vi "加标回收启动对话框.vi"(11 "测试模式":enum16{"水样测试", "平行样测试", "加标回收", "集成干预测试"}(ring)) -> (1 "流程参数":T1, 2 "启动参数":T2, 3 "check ？":bool)   [LabVIEW 2016, in "质控单元V4.lvlib"]
panel:
  in  "氟化物":bool caption="启用"
  in  "采配水":bool=TRUE
  in  "取消":bool
  in  "确认":bool
  in  "CODCr":bool caption="启用"
  in  "CODMn":bool caption="启用"
  in  "总氮":bool caption="启用"
  in  "总磷":bool caption="启用"
  in  "氨氮":bool caption="启用"
  # "请选择启动参数和流程"
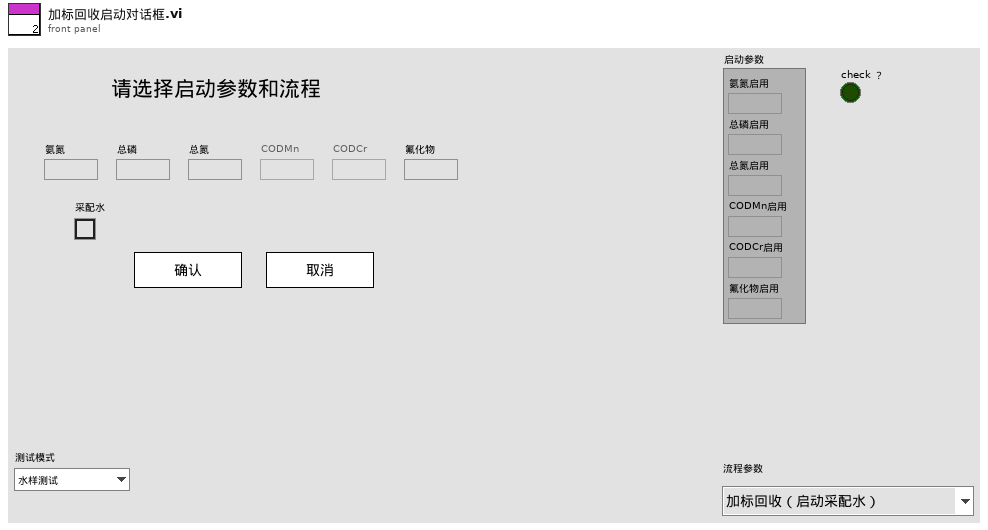
[diagram p1: front panel]
types:
  T1 = typedef "质控单元V4.lvlib/测试流程.ctl" = enum16{"加标回收（启动采配水）", "加标回收（不启动采配水）", "水样测试（启动采配水）", "水样测试（不启动采配水）", "平行样测试（启动采配水）", "平行样测试（不启动采配水）", "集成干预测试"}
  T2 = typedef "质控单元V4.lvlib/启动参数.ctl" = cluster{"氨氮启用":bool, "总磷启用":bool, "总氮启用":bool, "CODMn启用":bool, "CODCr启用":bool, "氟化物启用":bool}
  T3 = cluster{"氨氮":bool, "总磷":bool, "总氮":bool, "CODMn":bool, "CODCr":bool, "氟化物":bool}
  T4 = enum8{"Enabled", "Disabled", "Disabled and Grayed Out"}
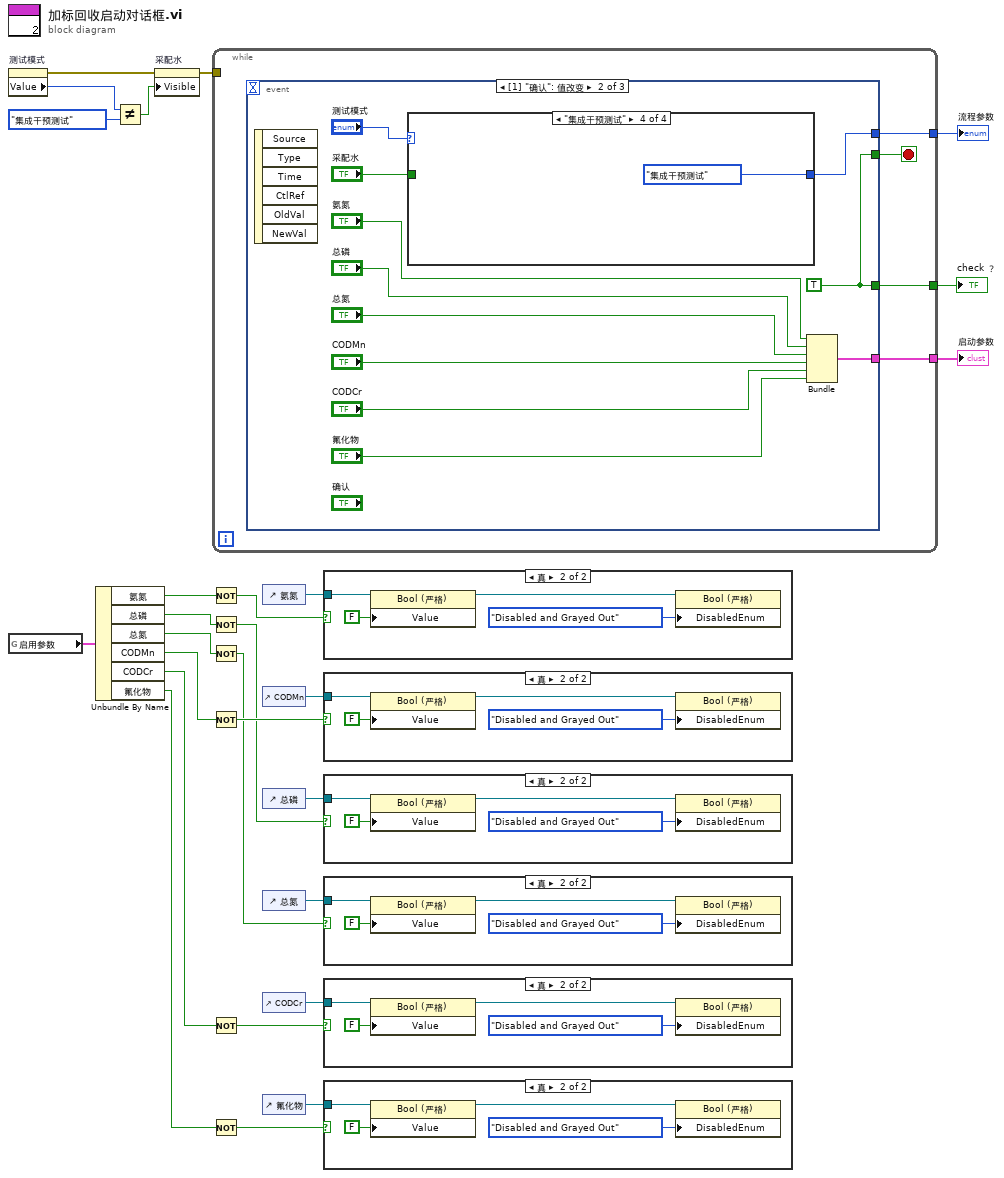
[diagram p0: block diagram]
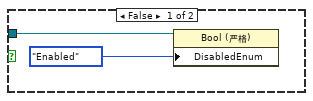
[diagram p2: hidden frame]
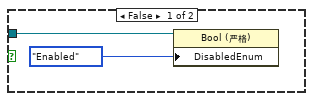
[diagram p3: hidden frame]
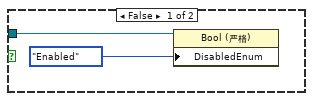
[diagram p4: hidden frame]
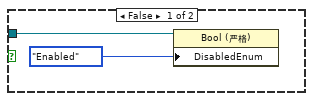
[diagram p5: hidden frame]
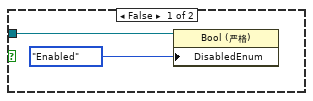
[diagram p6: hidden frame]
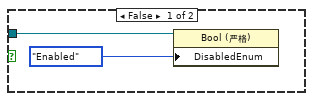
[diagram p7: hidden frame]
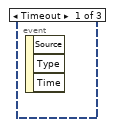
[diagram p8: hidden frame]
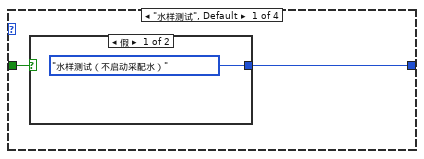
[diagram p9: hidden frame]
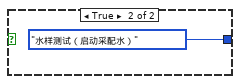
[diagram p10: hidden frame]
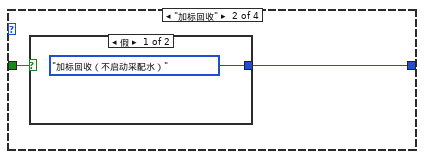
[diagram p11: hidden frame]
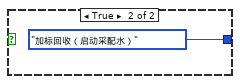
[diagram p12: hidden frame]
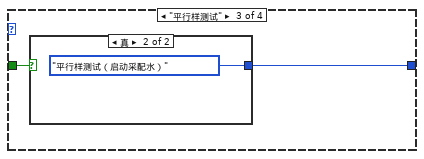
[diagram p13: hidden frame]
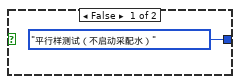
[diagram p14: hidden frame]
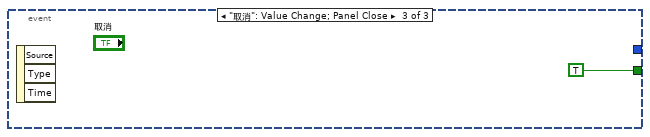
[diagram p15: hidden frame]
diagram:
  n1 = property on="测试模式" class="Enum (严格)"() -> (error out=w16:errorcluster, "Value"=w18:enum16{"水样测试", "平行样测试", "加标回收", "集成干预测试"})  [unwired: 2 in, 1 out]
  n2 = global read "ZK断电保存全局变量.vi" "启用参数"() -> (w19:T3)
  n3 = Unbundle By Name(w19) -> ("氨氮"=w10:bool, "总磷"=w11:bool, "总氮"=w9:bool, "CODMn"=w7:bool, "CODCr"=w8:bool, "氟化物"=w12:bool)
  n4 = Not Equal?(x=w18, y=enum16{"水样测试", "平行样测试", "加标回收", "集成干预测试"}."集成干预测试") -> (x != y?=w15:bool)
  n5 = property on="采配水" class="Bool (严格)"(error in=w16, "Visible"=w15) -> (error out=w14:errorcluster)  [unwired: 1 in, 1 out]
  n6 = Not(x=w10) -> (.not. x?=w1:bool)
  n7 = Not(x=w11) -> (.not. x?=w2:bool)
  n8 = Not(x=w9) -> (.not. x?=w3:bool)
  n9 = Not(x=w7) -> (.not. x?=w4:bool)
  n10 = Not(x=w8) -> (.not. x?=w5:bool)
  n11 = Not(x=w12) -> (.not. x?=w6:bool)
  n12 = while {
    tunnel: [w31] -> w27
    tunnel: [w29] -> w26
    tunnel: [w28] -> w25
    tunnel: w14 -> [_]
    stop <- w30 stop-if-true
    n13 = event shown="[1] \"确认\": 值改变" {
      selector: _ -> [_ _ _]
      dyn-events: _ -> [_ _ _]
      timeout: _ -> [_ _ _]
      tunnel: [_ w42 _] -> w31
      tunnel: [_ w42 TRUE] -> w30
      tunnel: [_ w36 _] -> w29
      tunnel: [_ w34 _] -> w28
      event Timeout {
        n14 = event-data() -> ()  [unwired: 1 in, 3 out]
      }
      event "确认": Value Change {
        w42 = TRUE
        n15 = event-data() -> ()  [unwired: 1 in, 6 out]
        n16 = case shown="\"集成干预测试\"" "测试模式" {
          tunnel: "采配水" -> [w44 w48 w52 _]
          tunnel: [w43 w47 w51 测试流程."集成干预测试" ("流程")] -> w34
          frame "水样测试", Default {
            n17 = case shown="假" w44 {
              tunnel: [测试流程."水样测试（不启动采配水）" ("流程") 测试流程."水样测试（启动采配水）" ("流程")] -> w43
              frame False {
              }
              frame True {
              }
            }
          }
          frame "加标回收" {
            n18 = case shown="假" w48 {
              tunnel: [测试流程."加标回收（不启动采配水）" ("流程") 测试流程."加标回收（启动采配水）" ("流程")] -> w47
              frame False {
              }
              frame True {
              }
            }
          }
          frame "平行样测试" {
            n19 = case shown="真" w52 {
              tunnel: [测试流程."平行样测试（不启动采配水）" ("流程") 测试流程."平行样测试（启动采配水）" ("流程")] -> w51
              frame False {
              }
              frame True {
              }
            }
          }
          frame "集成干预测试" {
          }
        }
        n20 = Bundle("氨氮"="氨氮", "总磷"="总磷", "总氮"="总氮", "CODMn"="CODMn", "CODCr"="CODCr", "氟化物"="氟化物") -> (w36:T3)  [unwired: 1 in]
      }
      event "取消": Value Change; Panel Close {
        n21 = event-data() -> ()  [unwired: 1 in, 3 out]
      }
    }
  }
  "check ？" <- w27
  "启动参数" <- w26
  "流程参数" <- w25
  n22 = control-ref of="氨氮"() -> (w24:refnum<vi>)
  n23 = control-ref of="CODMn"() -> (w21:refnum<vi>)
  n24 = control-ref of="总磷"() -> (w23:refnum<vi>)
  n25 = control-ref of="总氮"() -> (w22:refnum<vi>)
  n26 = control-ref of="CODCr"() -> (w20:refnum<vi>)
  n27 = control-ref of="氟化物"() -> (w13:refnum<vi>)
  n28 = case shown="真" w1 {
    tunnel: w24 -> [w57 w62]
    frame False {
      n29 = property class="Bool (严格)"(reference=w57, "DisabledEnum"=T4."Enabled" ("禁用")) -> ()  [unwired: 1 in, 2 out]
    }
    frame True {
      n30 = property class="Bool (严格)"(reference=w62, "Value"=FALSE ("值")) -> (reference out=w60:refnum<vi>)  [unwired: 1 in, 1 out]
      n31 = property class="Bool (严格)"(reference=w60, "DisabledEnum"=T4."Disabled and Grayed Out" ("禁用")) -> ()  [unwired: 1 in, 2 out]
    }
  }
  n32 = case shown="真" w4 {
    tunnel: w21 -> [w63 w68]
    frame False {
      n33 = property class="Bool (严格)"(reference=w63, "DisabledEnum"=T4."Enabled" ("禁用")) -> ()  [unwired: 1 in, 2 out]
    }
    frame True {
      n34 = property class="Bool (严格)"(reference=w68, "Value"=FALSE ("值")) -> (reference out=w66:refnum<vi>)  [unwired: 1 in, 1 out]
      n35 = property class="Bool (严格)"(reference=w66, "DisabledEnum"=T4."Disabled and Grayed Out" ("禁用")) -> ()  [unwired: 1 in, 2 out]
    }
  }
  n36 = case shown="真" w2 {
    tunnel: w23 -> [w69 w74]
    frame False {
      n37 = property class="Bool (严格)"(reference=w69, "DisabledEnum"=T4."Enabled" ("禁用")) -> ()  [unwired: 1 in, 2 out]
    }
    frame True {
      n38 = property class="Bool (严格)"(reference=w74, "Value"=FALSE ("值")) -> (reference out=w72:refnum<vi>)  [unwired: 1 in, 1 out]
      n39 = property class="Bool (严格)"(reference=w72, "DisabledEnum"=T4."Disabled and Grayed Out" ("禁用")) -> ()  [unwired: 1 in, 2 out]
    }
  }
  n40 = case shown="真" w3 {
    tunnel: w22 -> [w75 w80]
    frame False {
      n41 = property class="Bool (严格)"(reference=w75, "DisabledEnum"=T4."Enabled" ("禁用")) -> ()  [unwired: 1 in, 2 out]
    }
    frame True {
      n42 = property class="Bool (严格)"(reference=w80, "Value"=FALSE ("值")) -> (reference out=w78:refnum<vi>)  [unwired: 1 in, 1 out]
      n43 = property class="Bool (严格)"(reference=w78, "DisabledEnum"=T4."Disabled and Grayed Out" ("禁用")) -> ()  [unwired: 1 in, 2 out]
    }
  }
  n44 = case shown="真" w5 {
    tunnel: w20 -> [w81 w86]
    frame False {
      n45 = property class="Bool (严格)"(reference=w81, "DisabledEnum"=T4."Enabled" ("禁用")) -> ()  [unwired: 1 in, 2 out]
    }
    frame True {
      n46 = property class="Bool (严格)"(reference=w86, "Value"=FALSE ("值")) -> (reference out=w84:refnum<vi>)  [unwired: 1 in, 1 out]
      n47 = property class="Bool (严格)"(reference=w84, "DisabledEnum"=T4."Disabled and Grayed Out" ("禁用")) -> ()  [unwired: 1 in, 2 out]
    }
  }
  n48 = case shown="真" w6 {
    tunnel: w13 -> [w87 w92]
    frame False {
      n49 = property class="Bool (严格)"(reference=w87, "DisabledEnum"=T4."Enabled" ("禁用")) -> ()  [unwired: 1 in, 2 out]
    }
    frame True {
      n50 = property class="Bool (严格)"(reference=w92, "Value"=FALSE ("值")) -> (reference out=w90:refnum<vi>)  [unwired: 1 in, 1 out]
      n51 = property class="Bool (严格)"(reference=w90, "DisabledEnum"=T4."Disabled and Grayed Out" ("禁用")) -> ()  [unwired: 1 in, 2 out]
    }
  }
